vi "Carica nomi tabelle MEI NM.vi"(11 "Cluster INFO in":T1 {"IMPOSTAZIONI INGRESSI NM"."RPM" items=["TESTO", "TORSIOMETRO", "OTTICA"]; "IMPOSTAZIONI INGRESSI NM"."PRESSIONE\nMANDATA" items=["P1", "P2", "P3"]; "IMPOSTAZIONI INGRESSI NM"."PRESSIONE\nASPIRAZIONE" items=["P1", "P2", "P3"]; "IMPOSTAZIONI INGRESSI NM"."PORTATA\nSECONDARIA" items=["Q1", "Q2", "Q3"]; "IMPOSTAZIONI INGRESSI NM"."PORTATA\nPRINCIPALE" items=["Q1", "Q2", "Q3"]; "IMPOSTAZIONI INGRESSI UL"."RPM" items=["TESTO", "TORSIOMETRO", "OTTICA"]; "IMPOSTAZIONI INGRESSI UL"."PRESSIONE MANDATA" items=["P1", "P2", "P3"]; "IMPOSTAZIONI INGRESSI UL"."PRESSIONE ASPIRAZIONE" items=["P1", "P2", "P3"]; "IMPOSTAZIONI INGRESSI UL"."PORTATA SECONDARIA" items=["Q1", "Q2", "Q3"]; "IMPOSTAZIONI INGRESSI UL"."PORTATA PRINCIPALE" items=["Q1", "Q2", "Q3"]}) -> (1 "Risultati":string, 2 "Boolean":string, 3 "Dati":string)   [LabVIEW 2014]
uses:
  TypeDef/Cluster INFO.ctl
  TypeDef/WT SELECTION.ctl
  TypeDef/CH SELECTION.ctl
  TypeDef/ALIM SELECTION.ctl
  TypeDef/cDAQ Settings UL.ctl
  TypeDef/SETUP INGRESSO.ctl
  TypeDef/cDAQ Settings NM.ctl
panel:
  # "Freddo"
  # "Regime"
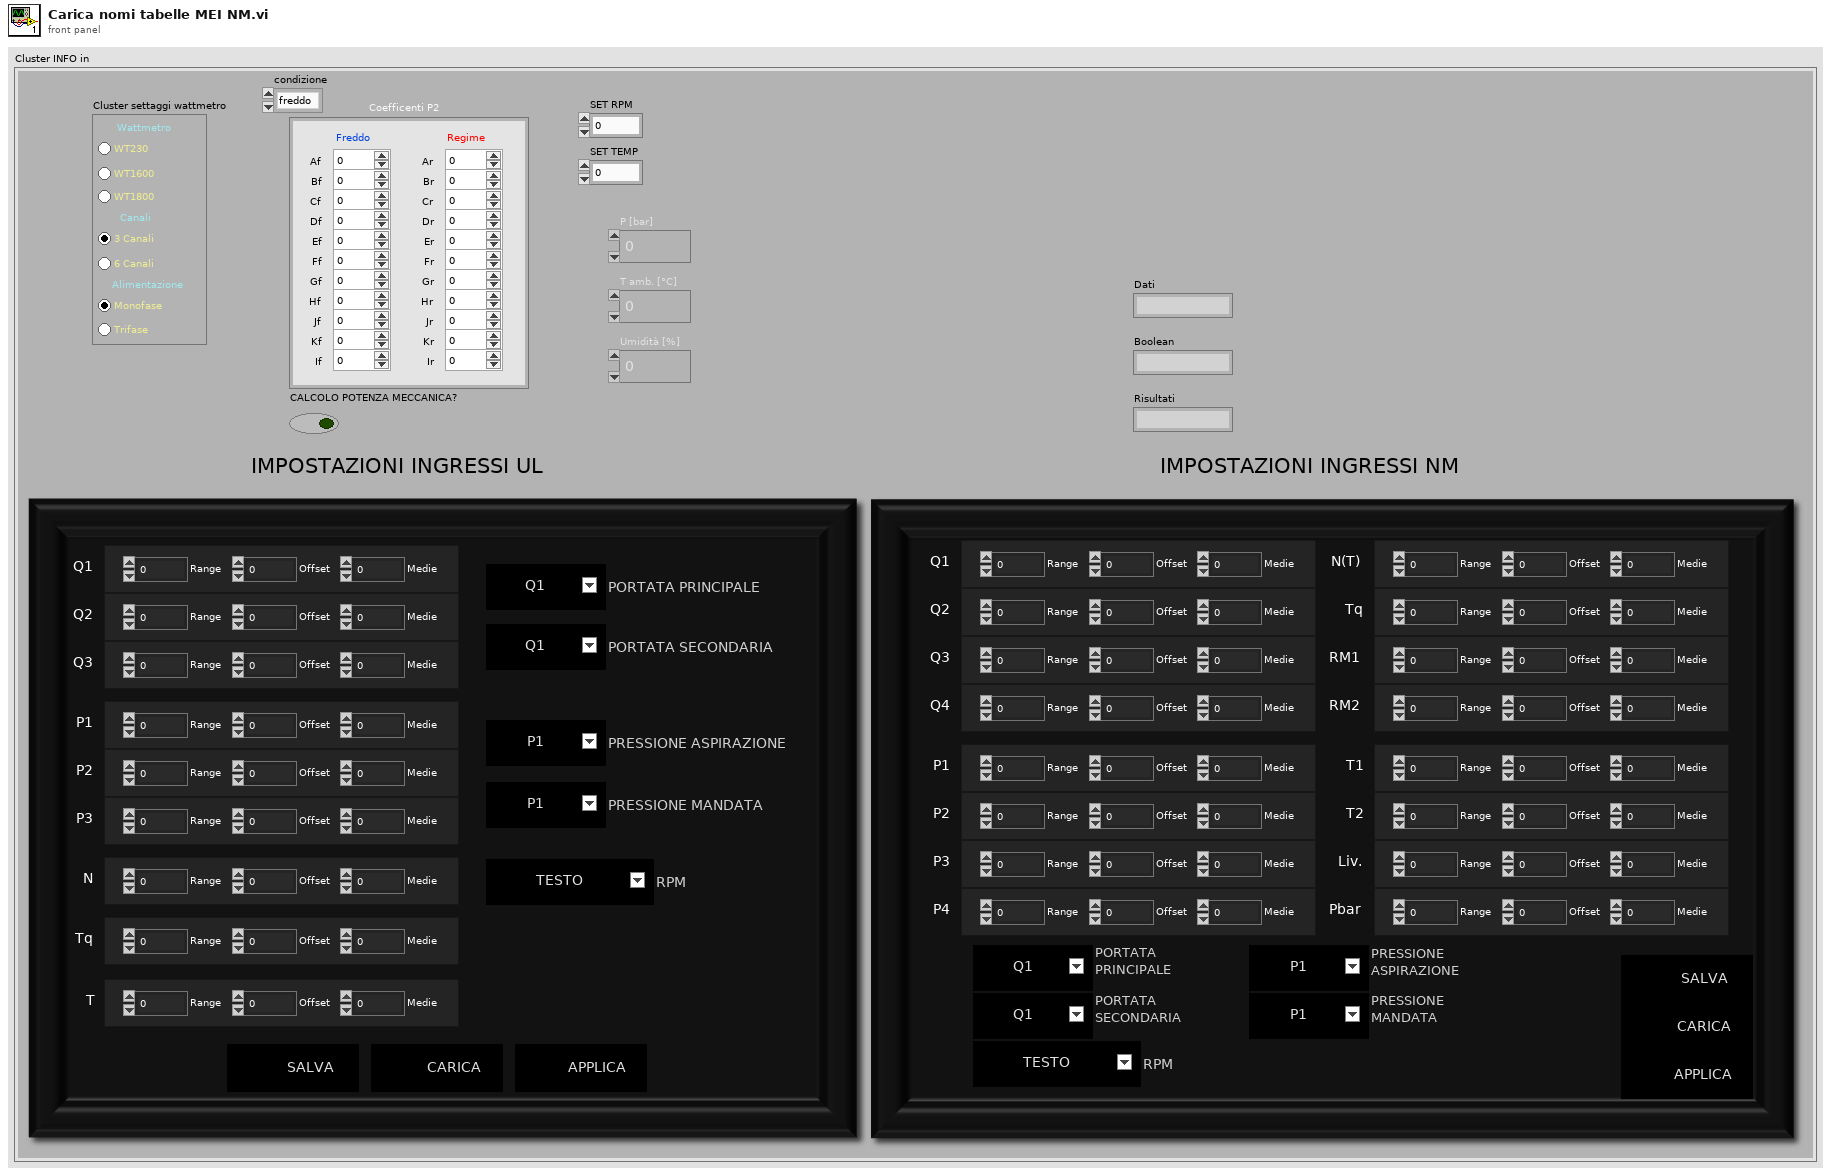
[diagram p1: front panel]
types:
  T1 = typedef "Cluster INFO.ctl" = cluster{"condizione":enum32{"freddo", "regime"}, "Coefficenti P2":cluster{"Af":dbl, "Bf":dbl, "Cf":dbl, "Df":dbl, "Ef":dbl, "Ff":dbl, "Gf":dbl, "Hf":dbl, "Jf":dbl, "Kf":dbl, "If":dbl, "Ar":dbl, "Br":dbl, "Cr":dbl, "Dr":dbl, "Er":dbl, "Fr":dbl, "Gr":dbl, "Hr":dbl, "Jr":dbl, "Kr":dbl, "Ir":dbl}, "Cluster settaggi wattmetro":cluster{"Wattmetro":T2, "Canali":T3, "Alimentazione":T4}, "CALCOLO POTENZA MECCANICA?":bool, "SET RPM":dbl, "SET TEMP":dbl, "IMPOSTAZIONI INGRESSI UL":T5, "IMPOSTAZIONI INGRESSI NM":T7, "Costanti collaudo":cluster{"P [bar]":dbl, "T amb. [°C]":dbl, "Umidità [%]":dbl}}
  T2 = typedef "WT SELECTION.ctl" = enum32{"No Selection", "Radio Selection 1", "Radio Selection 2", "Radio Selection 3"}
  T3 = typedef "CH SELECTION.ctl" = enum32{"Radio Selection 1", "Radio Selection 2"}
  T4 = typedef "ALIM SELECTION.ctl" = enum32{"Radio Selection 1", "Radio Selection 2"}
  T5 = typedef "cDAQ Settings UL.ctl" = cluster{"SALVA":bool, "CARICA":bool, "APPLICA":bool, "Q1":T6, "Q2":T6, "Q3":T6, "P1":T6, "P2":T6, "P3":T6, "N":T6, "Tq":T6, "T":T6, "PORTATA PRINCIPALE":u16, "PORTATA SECONDARIA":u16, "PRESSIONE ASPIRAZIONE":u16, "PRESSIONE MANDATA":u16, "RPM":u16}
  T6 = typedef "SETUP INGRESSO.ctl" = cluster{"Range":dbl, "Offset":dbl, "Medie":u8}
  T7 = typedef "cDAQ Settings NM.ctl" = cluster{"SALVA":bool, "CARICA":bool, "APPLICA":bool, "Q1":T6, "Q2":T6, "Q3":T6, "Q4":T6, "N(T)":T6, "Tq":T6, "RM1":T6, "RM2":T6, "P1":T6, "P2":T6, "P3":T6, "P4":T6, "T1":T6, "T2":T6, "Liv.":T6, "Pbar":T6, "PORTATA\nPRINCIPALE":u16, "PORTATA\nSECONDARIA":u16, "PRESSIONE\nASPIRAZIONE":u16, "PRESSIONE\nMANDATA":u16, "RPM":u16}
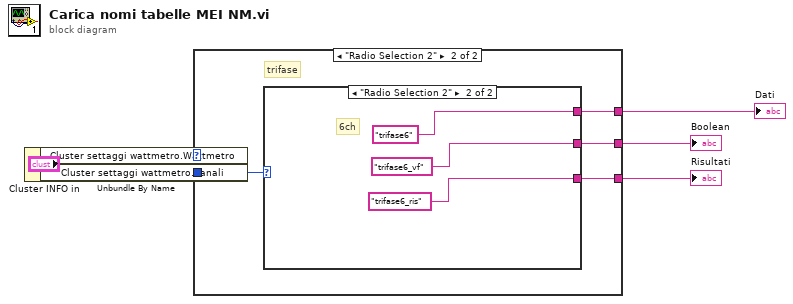
[diagram p0: block diagram]
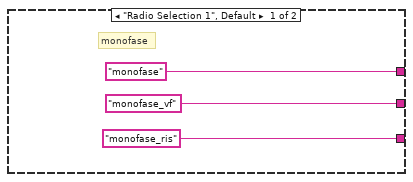
[diagram p2: hidden frame]
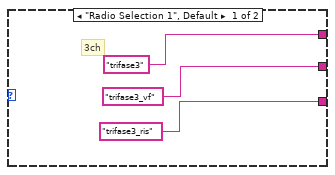
[diagram p3: hidden frame]
diagram:
  n1 = Unbundle By Name("Cluster INFO in") -> ("Cluster settaggi wattmetro.Wattmetro"=w5:T2, "Cluster settaggi wattmetro.Canali"=w6:T3)
  n2 = case shown="\"Radio Selection 2\"" w5 {
    tunnel: ["monofase" w13] -> w3
    tunnel: ["monofase_vf" w12] -> w2
    tunnel: ["monofase_ris" w11] -> w1
    tunnel: w6 -> [_ w10]
    frame "Radio Selection 1", Default {
      # "monofase"
    }
    frame "Radio Selection 2" {
      # "trifase"
      n3 = case shown="\"Radio Selection 2\"" w10 {
        tunnel: ["trifase3" "trifase6"] -> w13
        tunnel: ["trifase3_vf" "trifase6_vf"] -> w12
        tunnel: ["trifase3_ris" "trifase6_ris"] -> w11
        frame "Radio Selection 1", Default {
          # "3ch"
        }
        frame "Radio Selection 2" {
          # "6ch"
        }
      }
    }
  }
  "Dati" <- w3
  "Boolean" <- w2
  "Risultati" <- w1
